vi "clear Session Data.vi"(0 "Session In":refnum<class "FPGA Session.lvclass">, 11 "error in":errorcluster) -> (4 "Session Out":refnum<class "FPGA Session.lvclass">, 15 "error out":errorcluster)   [LabVIEW 2016, in "FPGA Session.lvclass"]
doc: "OVERRIDE VI\nPlaceholder for decendant classes to clear session information and close references."
uses:
  FPGA Session.lvclass
  FPGA Session.lvclass/FPGA Session.ctl
  <vilib>/FPGAPlugInAG/cRIO-9081/niLvFpga_Close_cRIO-9081.vi
  <vilib>/rvi/interface/nirviCloseFPGA/nirviCloseFPGA.xnode
  FPGA Ref.ctl
  FPGA Bitfiles/serverv4.lvbitx
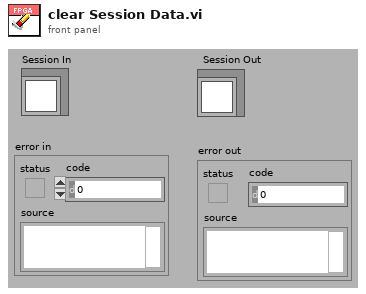
[diagram p1: front panel]
types:
  T1 = typedef "FPGA Ref.ctl" = refnum<k20>
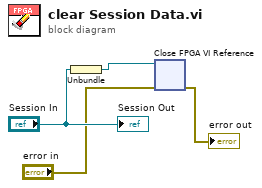
[diagram p0: block diagram]
diagram:
  n1 = Unbundle("Session In") -> (w3:T1)
  n2 = xnode "Close FPGA VI Reference"("FPGA VI Reference In"=w3, "error in"="error in") -> ("error out"=→"error out":errorcluster)
  "Session Out" <- "Session In"
